vi "Create error queue.vi"(8 "Error in":errorcluster caption="Error in (no error)") -> (0 "Error out":errorcluster)   [LabVIEW 2020]
uses:
  Error log.ctl
panel:
  out "queue out":refnum<queue>
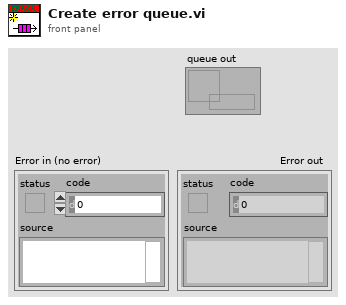
[diagram p1: front panel]
types:
  T1 = typedef "Error log.ctl" = cluster{timestamp, string[], "error in (no error)":errorcluster}
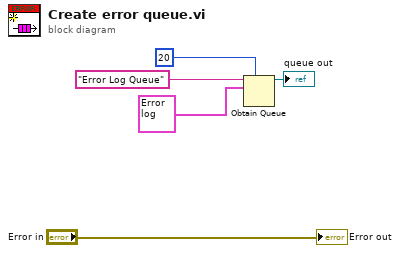
[diagram p0: block diagram]
diagram:
  n1 = Obtain Queue(max queue size (-1, unlimited)=20, name (unnamed)="Error Log Queue", element data type=T1 {timestamp(0 s since 1904-01-01), [], "error in (no error)"={"status"=FALSE, "code"=0, "source"=""}}) -> (queue out=→"queue out":refnum<queue>)  [unwired: 2 in, 2 out]
  "Error out" <- "Error in"
